vi "Tektronix cursor Read.vi"(8 "error in (no error)":errorcluster, 11 "Datos Osciloscopio":T1={"Sesión Visa Osciloscopio"="Tektronix_TDS2012C", "Tipo de Adquisición"=enum."Voltaje Pico Pico", "Canal a Utilizar"=enum."Canal 1", "Parametros de Adquisición"=enum."Una Muestra", "Número Promedio"=0} {"Número Promedio" min=2 max=20}) -> (0 "error out":errorcluster, 2 "Dato":string, 3 "CH1":dbl)   [LabVIEW 2020]
uses:
  Type Definitions/datos osciloscopio.ctl
panel:
  out "CH2":dbl
  out "Dato CH2":string
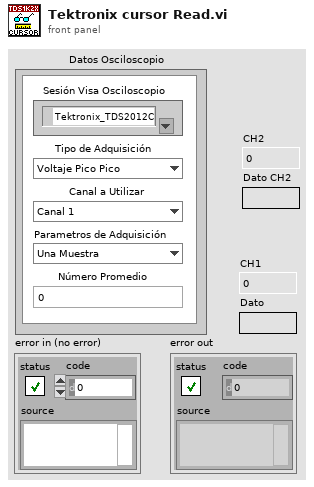
[diagram p1: front panel]
types:
  T1 = typedef "datos osciloscopio.ctl" = cluster{"Sesión Visa Osciloscopio":refnum<visa-resource-name>, "Tipo de Adquisición":enum16{"Voltaje Pico Pico", "Voltaje RMS", "Cursor Tiempo"}, "Canal a Utilizar":enum16{"Canal 1", "Canal 2", "Canal 1 y 2"}, "Parametros de Adquisición":enum16{"Una Muestra", "Promedio"}, "Número Promedio":i32}
  T2 = enum16{"Voltaje Pico Pico", "Voltaje RMS", "Cursor Tiempo"}
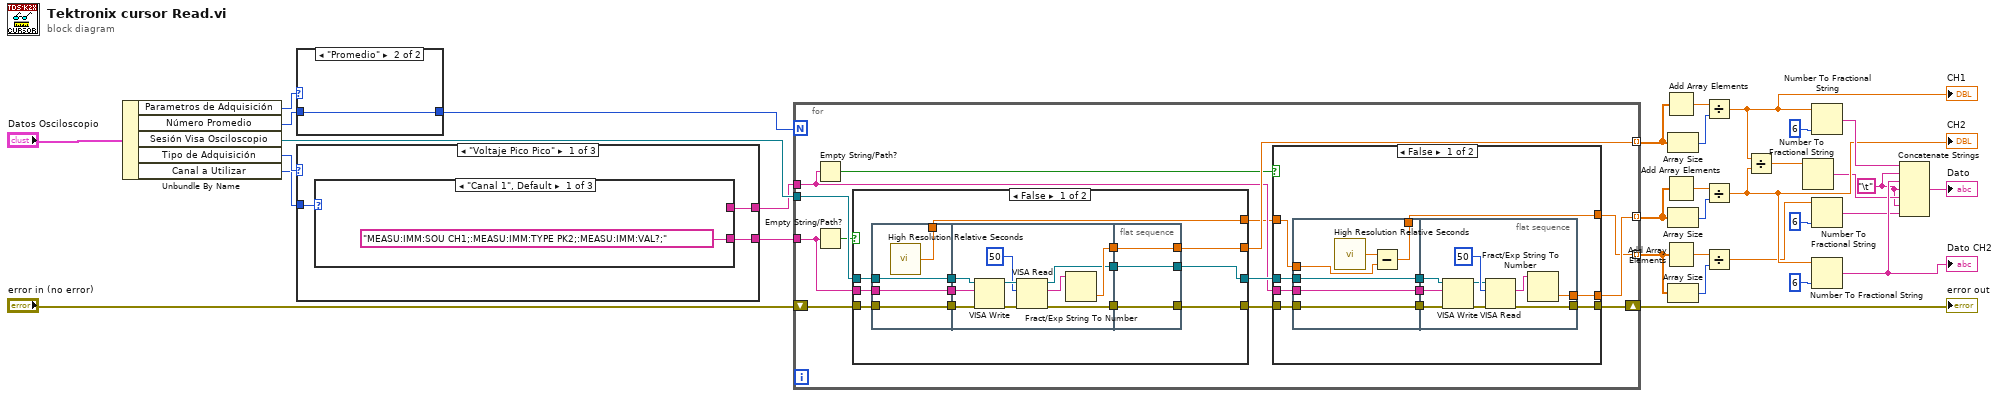
[diagram p0: block diagram]
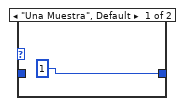
[diagram p2: hidden frame]
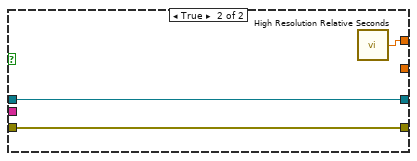
[diagram p3: hidden frame]
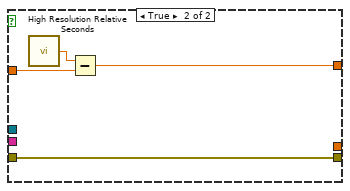
[diagram p4: hidden frame]
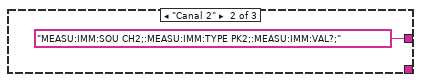
[diagram p5: hidden frame]
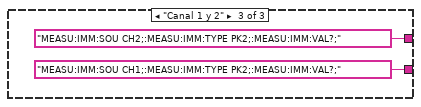
[diagram p6: hidden frame]
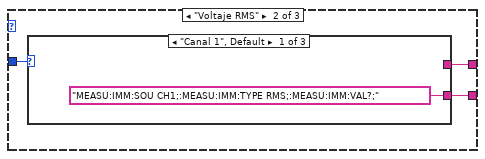
[diagram p7: hidden frame]
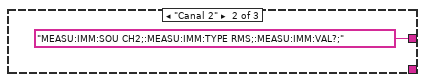
[diagram p8: hidden frame]
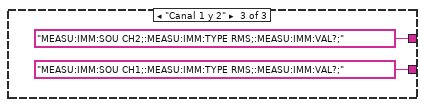
[diagram p9: hidden frame]
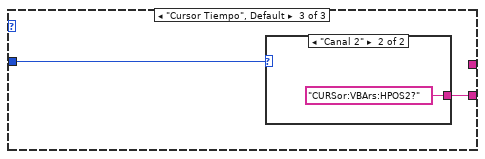
[diagram p10: hidden frame]
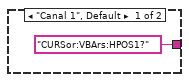
[diagram p11: hidden frame]
diagram:
  w4 = "\t"
  n1 = Unbundle By Name("Datos Osciloscopio") -> ("Parametros de Adquisición"=w25:enum16{"Una Muestra", "Promedio"}, "Número Promedio"=w24:i32, "Sesión Visa Osciloscopio"=w28:refnum<visa-resource-name>, "Tipo de Adquisición"=w30:T2, "Canal a Utilizar"=w29:enum16{"Canal 1", "Canal 2", "Canal 1 y 2"})
  n2 = case shown="\"Promedio\"" w25 {
    tunnel: w24 -> [_ w35]
    tunnel: [1 w35] -> w26
    frame "Una Muestra", Default {
    }
    frame "Promedio" {
    }
  }
  n3 = case shown="\"Voltaje Pico Pico\"" w30 {
    tunnel: [w38 w45 w51] -> w33
    tunnel: w29 -> [w37 w44 w50]
    tunnel: [w36 w43 _] -> w19
    frame "Voltaje Pico Pico" {
      n4 = case shown="\"Canal 1\", Default" w37 {
        tunnel: ["MEASU:IMM:SOU CH1;:MEASU:IMM:TYPE PK2;:MEASU:IMM:VAL?;" ("write buffer") _ "MEASU:IMM:SOU CH1;:MEASU:IMM:TYPE PK2;:MEASU:IMM:VAL?;" ("write buffer")] -> w38
        tunnel: [_ "MEASU:IMM:SOU CH2;:MEASU:IMM:TYPE PK2;:MEASU:IMM:VAL?;" ("write buffer") "MEASU:IMM:SOU CH2;:MEASU:IMM:TYPE PK2;:MEASU:IMM:VAL?;" ("write buffer")] -> w36
        frame "Canal 1", Default {
        }
        frame "Canal 2" {
        }
        frame "Canal 1 y 2" {
        }
      }
    }
    frame "Voltaje RMS" {
      n5 = case shown="\"Canal 1\", Default" w44 {
        tunnel: ["MEASU:IMM:SOU CH1;:MEASU:IMM:TYPE RMS;:MEASU:IMM:VAL?;" ("write buffer") _ "MEASU:IMM:SOU CH1;:MEASU:IMM:TYPE RMS;:MEASU:IMM:VAL?;" ("write buffer")] -> w45
        tunnel: [_ "MEASU:IMM:SOU CH2;:MEASU:IMM:TYPE RMS;:MEASU:IMM:VAL?;" ("write buffer") "MEASU:IMM:SOU CH2;:MEASU:IMM:TYPE RMS;:MEASU:IMM:VAL?;" ("write buffer")] -> w43
        frame "Canal 1", Default {
        }
        frame "Canal 2" {
        }
        frame "Canal 1 y 2" {
        }
      }
    }
    frame "Cursor Tiempo", Default {
      n6 = case shown="\"Canal 2\"" w50 {
        tunnel: ["CURSor:VBArs:HPOS1?" ("write buffer") "CURSor:VBArs:HPOS2?" ("write buffer")] -> w51
        frame "Canal 1", Default {
        }
        frame "Canal 2" {
        }
      }
    }
  }
  n7 = for {
    N: w26 -> [_]
    tunnel: w33 -> [w57]
    tunnel: w28 -> [w66]
    shift-right: [w60] -> w32
    shift-left: "error in (no error)" -> [w65]
    tunnel: [w64] -> w23 mode=indexing
    tunnel: w19 -> [w62]
    tunnel: [w59] -> w15 mode=indexing
    tunnel: [w54] -> w5 mode=indexing
    n8 = Empty String/Path?(string/path=w62) -> (empty?=w58:bool)
    n9 = Empty String/Path?(string/path=w57) -> (empty?=w56:bool)
    n10 = case shown="False" w56 {
      tunnel: w66 -> [w79 w98]
      tunnel: w65 -> [w78 w99]
      tunnel: [w77 _] -> w64
      tunnel: [w76 w98] -> w63
      tunnel: [w75 w99] -> w61
      tunnel: w57 -> [w74 _]
      tunnel: [w67 w97] -> w55
      frame False {
        n11 = flat-sequence {
          tunnel: w74 -> [w81]
          tunnel: w78 -> [w82]
          tunnel: w79 -> [w83]
          tunnel: [w83] -> w73
          tunnel: [w82] -> w72
          tunnel: [w81] -> w71
          tunnel: [w80] -> w67
          tunnel: w73 -> [w89]
          tunnel: w72 -> [w88]
          tunnel: w71 -> [w84]
          tunnel: [w87] -> w70
          tunnel: [w86] -> w69
          tunnel: [w85] -> w68
          tunnel: [w94] -> w75
          tunnel: [w95] -> w76
          tunnel: [w96] -> w77
          tunnel: w70 -> [w96]
          tunnel: w69 -> [w95]
          tunnel: w68 -> [w94]
          frame #0 {
            n12 = call <vilib>:"High Resolution Relative Seconds.vi"() -> ("relative seconds"=w80:dbl)
          }
          frame #1 {
            n13 = VISA Write(VISA resource name=w89, write buffer=w84, error in (no error)=w88) -> (VISA resource name out=w93:refnum<visa-resource-name>, error out=w92:errorcluster)  [unwired: 1 out]
            n14 = VISA Read(VISA resource name=w93, byte count=u32 50, error in (no error)=w92) -> (VISA resource name out=w86:refnum<visa-resource-name>, read buffer=w90:string, error out=w85:errorcluster)  [unwired: 1 out]
            n15 = Fract/Exp String To Number(string=w90) -> (number=w87:dbl)  [unwired: 3 in, 1 out]
          }
          frame #2 {
          }
        }
      }
      frame True {
        n16 = call <vilib>:"High Resolution Relative Seconds.vi"() -> ("relative seconds"=w97:dbl)
      }
    }
    n17 = case shown="False" w58 {
      tunnel: w63 -> [w109 _]
      tunnel: w62 -> [w108 _]
      tunnel: w61 -> [w107 w128]
      tunnel: [w106 w128] -> w60
      tunnel: [w105 _] -> w59
      tunnel: w55 -> [w101 w126]
      tunnel: [w100 w125] -> w54
      frame False {
        n18 = flat-sequence {
          tunnel: w107 -> [w113]
          tunnel: w108 -> [w114]
          tunnel: w109 -> [w115]
          tunnel: [w115] -> w104
          tunnel: [w114] -> w103
          tunnel: [w113] -> w102
          tunnel: w101 -> [w111]
          tunnel: [w110] -> w100
          tunnel: [w117] -> w106
          tunnel: [w116] -> w105
          tunnel: w104 -> [w120]
          tunnel: w103 -> [w119]
          tunnel: w102 -> [w118]
          frame #0 {
            n19 = call <vilib>:"High Resolution Relative Seconds.vi"() -> ("relative seconds"=w112:dbl)
            n20 = Subtract(x=w112, y=w111) -> (x-y=w110:dbl)
          }
          frame #1 {
            n21 = VISA Write(VISA resource name=w120, write buffer=w119, error in (no error)=w118) -> (VISA resource name out=w121:refnum<visa-resource-name>, error out=w122:errorcluster)  [unwired: 1 out]
            n22 = VISA Read(VISA resource name=w121, byte count=u32 50, error in (no error)=w122) -> (read buffer=w124:string, error out=w117:errorcluster)  [unwired: 2 out]
            n23 = Fract/Exp String To Number(string=w124) -> (number=w116:dbl)  [unwired: 3 in, 1 out]
          }
        }
      }
      frame True {
        n24 = call <vilib>:"High Resolution Relative Seconds.vi"() -> ("relative seconds"=w127:dbl)
        n25 = Subtract(x=w127, y=w126) -> (x-y=w125:dbl)
      }
    }
  }
  "error out" <- w32
  n26 = Add Array Elements(numeric array=w23) -> (sum=w22:dbl)
  n27 = Add Array Elements(numeric array=w15) -> (sum=w16:dbl)
  n28 = Add Array Elements(numeric array=w5) -> (sum=w6:dbl)
  n29 = Array Size(array=w23) -> (size(s)=w21:i32)
  n30 = Array Size(array=w15) -> (size(s)=w17:i32)
  n31 = Array Size(array=w5) -> (size(s)=w7:i32)
  n32 = Divide(x=w22, y=w21) -> (x/y=w11:dbl)
  "CH1" <- w11
  n33 = Divide(x=w16, y=w17) -> (x/y=w10:dbl)
  "CH2" <- w10
  n34 = Divide(x=w6, y=w7) -> (x/y=w2:dbl)
  n35 = Divide(x=w11, y=w10) -> (x/y=w9:dbl)
  n36 = Number To Fractional String(number=w9) -> (F-format string=w8:string)  [unwired: 3 in]
  n37 = Number To Fractional String(number=w11, precision (6)=i16 6) -> (F-format string=w14:string)  [unwired: 2 in]
  n38 = Number To Fractional String(number=w2, precision (6)=i16 6) -> (F-format string=w1:string)  [unwired: 2 in]
  n39 = Number To Fractional String(number=w10, precision (6)=i16 6) -> (F-format string=w13:string)  [unwired: 2 in]
  "Dato CH2" <- w13
  n40 = Concatenate Strings(w14, w4, w13, w4, w8, w4, w1) -> (→"Dato":string)
